vi "ADAM Server Alive.vi"() -> (2 "Server time":dbl format="%.2f", 3 "Difference":dbl format="%.2f", 4 "error Out":errorcluster)   [LabVIEW 2017]
doc: "This is an example of using features of the VI Server as a client. It shows how you might browse from one or more applications that may be exporting data from one or more data stations. \n\nThe example shows how to query a server for its list of exported VIs, how to get references to the VIs, and how call them with the Call By Reference function."
uses:
  Anemometry/Anemometry Sub Vis/Globals/Preference_global.vi
panel:
  out "Iterations":i32
  in  "trivial.vi type":refnum<vi>
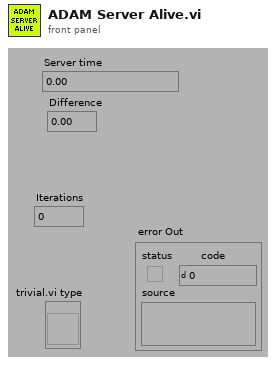
[diagram p1: front panel]
types:
  T1 = typedef "Server_Comms.ctl" = enum16{"Server Link Healthy", "Do Not Link To Server"}
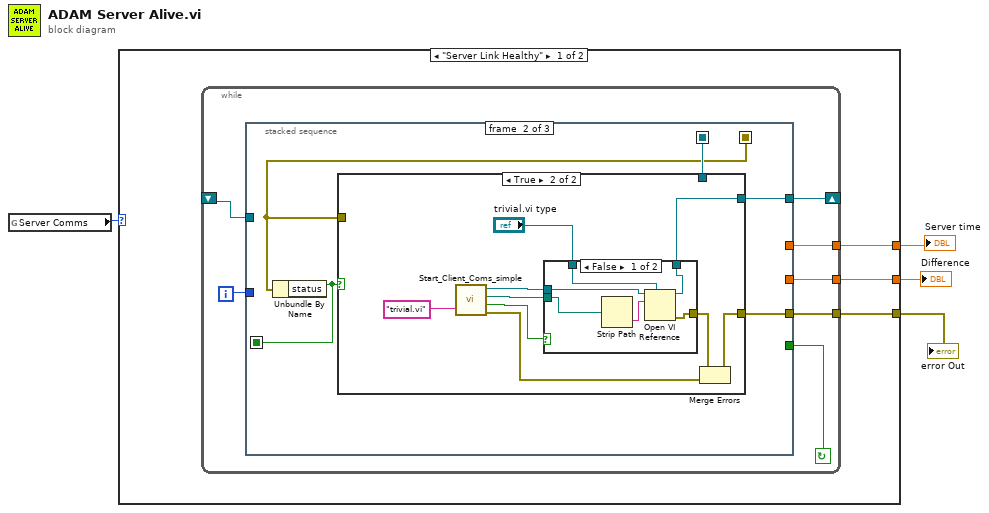
[diagram p0: block diagram]
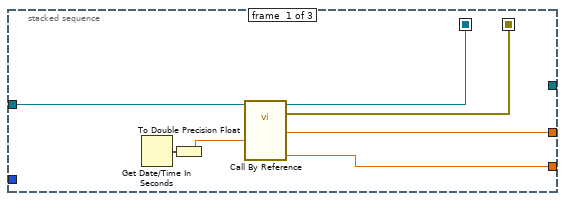
[diagram p2: hidden frame]
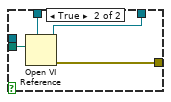
[diagram p4: hidden frame]
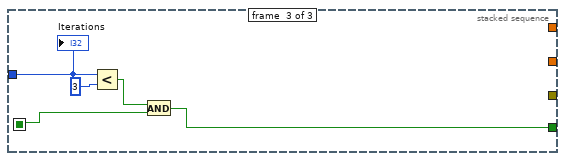
[diagram p5: hidden frame]
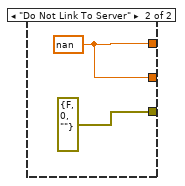
[diagram p6: hidden frame]
diagram:
  n1 = global read "Preference_global.vi" "Server Comms"() -> (w4:T1)
  n2 = case shown="\"Server Link Healthy\"" w4 {
    tunnel: [w7 errorcluster {"status"=FALSE, "code"=0, "source"=""}] -> w3
    tunnel: [w6 w53] -> w2
    tunnel: [w5 w53] -> w1
    frame "Server Link Healthy" {
      n3 = while {
        tunnel: [w10] -> w7
        shift-left: _ -> [w14]
        shift-right: [w13] -> _
        tunnel: [w9] -> w6
        tunnel: [w8] -> w5
        i -> [w12]
        stop <- w11 continue-if-true
        n4 = stacked-sequence {
          seq-local: [w18 _ _] -> [_ w25 _]
          seq-local: [w20 _ _] -> [_ w22 _]
          seq-local: [_ w24 _] -> [_ _ w49]
          tunnel: w14 -> [w19 _ _]
          tunnel: [_ w26 _] -> w13
          tunnel: w12 -> [_ _ w50]
          tunnel: [_ _ w48] -> w11
          tunnel: [_ w23 _] -> w10
          tunnel: [w16 _ _] -> w9
          tunnel: [w15 _ _] -> w8
          frame #0 {
            n5 = Get Date/Time In Seconds() -> (seconds since 1Jan1904=w17:timestamp)
            n6 = To Double Precision Float(number=w17) -> (double precision float=w21:dbl)
            n7 = call-by-ref "?"(reference=w19, "Client time"=w21) -> (reference out=w18:refnum<vi>, error out=w20:errorcluster, "Server time"=w16:dbl, "Difference"=w15:dbl)  [unwired: 1 in]
          }
          frame #1 {
            n8 = Unbundle By Name(w22) -> ("status"=w24:bool)
            n9 = case shown="True" w24 {
              tunnel: [w28 w36] -> w26
              tunnel: w25 -> [w28 _]
              tunnel: [w27 w30] -> w23
              tunnel: w22 -> [w27 _]
              frame False {
              }
              frame True {
                n10 = call "Start_Client_Coms_simple.vi"("VI name to run on server"="trivial.vi") -> ("LabVIEW application reference"=w35:refnum<vi>, "Checked VI name"=w34:path, "Local Call"=w33:bool, "output cluster"=w29:errorcluster)  [unwired: 1 in]
                n11 = case shown="False" w33 {
                  tunnel: [w40 w47] -> w36
                  tunnel: "trivial.vi type" -> [w39 w46]
                  tunnel: w34 -> [w41 w45]
                  tunnel: w35 -> [w38 _]
                  tunnel: [w42 w44] -> w31
                  frame False {
                    n12 = Strip Path(path=w41) -> (name=w43:string)  [unwired: 1 out]
                    n13 = Open VI Reference(type specifier VI Refnum (for type only)=w39, application reference (local)=w38, vi path=w43) -> (vi reference=w40:refnum<vi>, error out=w42:errorcluster)  [unwired: 1 in, 2 out]
                  }
                  frame True {
                    n14 = Open VI Reference(type specifier VI Refnum (for type only)=w46, vi path=w45) -> (vi reference=w47:refnum<vi>, error out=w44:errorcluster)  [unwired: 1 in, 3 out]
                  }
                }
                n15 = Merge Errors(w31, w29) -> (w30:errorcluster)
              }
            }
          }
          frame #2 {
            n16 = Less?(x=w50, y=3) -> (x < y?=w52:bool)
            n17 = And(x=w52, y=w49) -> (x .and. y?=w48:bool)
            "Iterations" <- w50
          }
        }
      }
    }
    frame "Do Not Link To Server" {
      w53 = nan ("Server time")
    }
  }
  "error Out" <- w3
  "Server time" <- w2
  "Difference" <- w1
